vi "Variant to DBL.vi"(8 "error in":errorcluster, 9 "Variant Value":variant) -> (0 "error out":errorcluster, 1 "DBL Value":dbl)   [LabVIEW 2018, in "Tag Engine.lvlib"]
doc: "Attempt to convert a variant value to Double precision floating point.\n\nThis might work for the following types:\n- Boolean: T=1.0, F=0.0\n- Unsigned Integer: U8..U64, Enum U8..U64\n- Signed Integer: I8..I64\n- Floating Point: SGL, DBL, EXT\n- String: Assuming Frac/Expr string using dot decimal place.\n- Timestamp: Converts to time in seconds.\n\nUnsupported types will return NaN for the value, without producing an error."
uses:
  Tag Engine.lvlib
  <vilib>/Utility/Data Type/NI_Data Type.lvlib
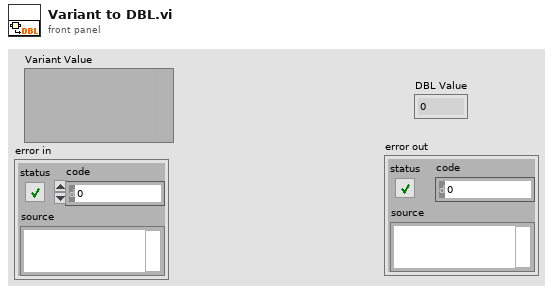
[diagram p1: front panel]
types:
  T1 = typedef "NI_Data Type.lvlib/Data Type.ctl" = enum8{"Invalid Type", "Void", "I8", "I16", "I32", "I64", "U8", "U16", "U32", "U64", "Single Float", "Double Float", "Extended Float", "Single Complex", "Double Complex", "Extended Complex", "Enum U8", "Enum U16", "Enum U32", "Enum U64", "Single Float With Unit", "Double Float With Unit", "Extended Float With Unit", "Single Complex with Unit", "Double Complex with Unit", "Extended Complex with Unit", "Boolean", "String", "Path", "Picture", "Tag", "Array", "Cluster", "Variant", "LV Variant", "Waveform", "Timestamp", "Digital Waveform", "Digital Data", "ExpressData", "Refnum", "External Data", "VI", "Poly VI", "LabVIEW Class Instance", "Fixed Point"}
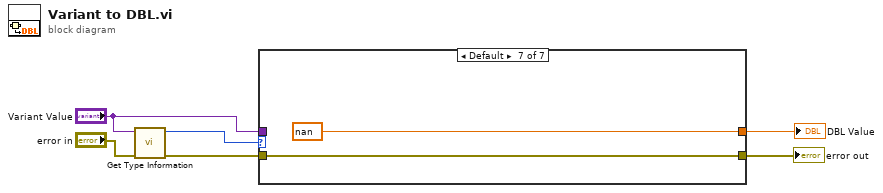
[diagram p0: block diagram]
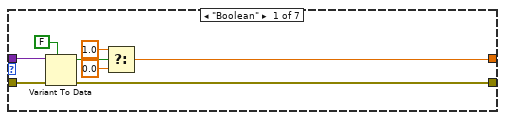
[diagram p2: hidden frame]
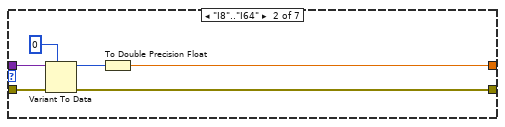
[diagram p3: hidden frame]
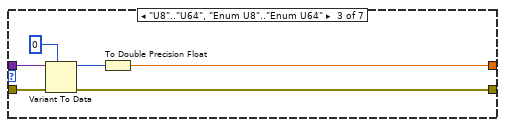
[diagram p4: hidden frame]
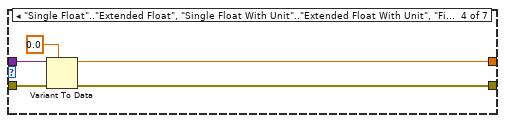
[diagram p5: hidden frame]
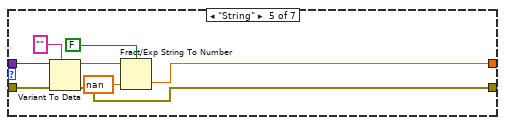
[diagram p6: hidden frame]
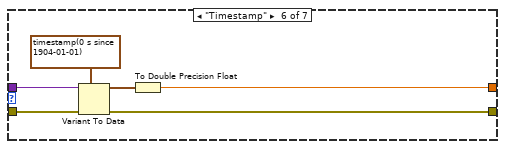
[diagram p7: hidden frame]
diagram:
  n1 = call <vilib>:"Get Type Information.vi"("error in (no error)"="error in", "Variant"="Variant Value") -> ("error out"=w2:errorcluster, "Type"=w4:T1)  [unwired: 5 in, 3 out]
  n2 = case shown="Default" w4 {
    tunnel: "Variant Value" -> [w14 w20 w26 w31 w38 w45 _]
    tunnel: [w9 w17 w23 w29 w34 w41 nan ("f")] -> w6
    tunnel: [w8 w15 w21 w27 w32 w40 w46] -> w5
    tunnel: w2 -> [w7 w16 w22 w28 w33 w44 w46]
    frame "Boolean" {
      n3 = Variant To Data(error in=w7, type=FALSE, Variant=w14) -> (data=w12:bool, error out=w8:errorcluster)
      n4 = Select(t=1.0, s=w12, f=0.0) -> (s? t:f=w9:dbl)
    }
    frame "I8".."I64" {
      n5 = Variant To Data(error in=w16, type=i64 0, Variant=w20) -> (data=w18:i64, error out=w15:errorcluster)
      n6 = To Double Precision Float(number=w18) -> (double precision float=w17:dbl)
    }
    frame "U8".."U64", "Enum U8".."Enum U64" {
      n7 = Variant To Data(error in=w22, type=u64 0, Variant=w26) -> (data=w24:u64, error out=w21:errorcluster)
      n8 = To Double Precision Float(number=w24) -> (double precision float=w23:dbl)
    }
    frame "Single Float".."Extended Float", "Single Float With Unit".."Extended Float With Unit", "Fixed Point" {
      n9 = Variant To Data(error in=w28, type=0.0, Variant=w31) -> (data=w29:dbl, error out=w27:errorcluster)
    }
    frame "String" {
      n10 = Variant To Data(error in=w33, type="", Variant=w38) -> (data=w36:string, error out=w32:errorcluster)
      n11 = Fract/Exp String To Number(use system decimal point (T)=FALSE, string=w36, default (0 dbl)=nan ("default (0 DBL)")) -> (number=w34:dbl)  [unwired: 1 in, 1 out]
    }
    frame "Timestamp" {
      n12 = Variant To Data(error in=w44, type=timestamp(0 s since 1904-01-01), Variant=w45) -> (data=w42:timestamp, error out=w40:errorcluster)
      n13 = To Double Precision Float(number=w42) -> (double precision float=w41:dbl)
    }
    frame Default {
    }
  }
  "DBL Value" <- w6
  "error out" <- w5
